vi "start_can_master.vi"(10 "br":u8, 11 "net":u8) -> (3 "return":i16)   [LabVIEW 2011]
uses:
  canopen_dll_master.dll
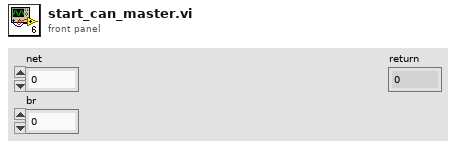
[diagram p1: front panel]
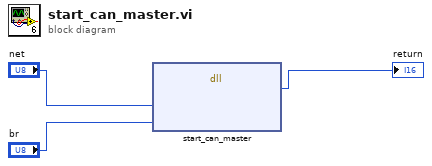
[diagram p0: block diagram]
diagram:
  n1 = dll-call lib="canopen_dll_master.dll" fn="start_can_master"("net"="net", "br"="br") -> ("return type"=→"return":i16)  [unwired: 5 in, 2 out]
